vi "Template - Error Handler.vi"(7 "Command (Check for Error)":T5=enum."Check", 8 "error in (no error)":errorcluster, 11 "QU Ref cluster":T4) -> (0 "error out":errorcluster)   [LabVIEW 2012]
doc: "This VI is the main VI for the error module. This VI will shutdown the application cleanly if an error occurs.\n\nThe errors can then be reported back."
uses:
  Navistar Library/Controls/TypeDef_Error_Command_enum.ctl
  TypeDef - Template - Q1 Ref.ctl
  TypeDef - Template - Queue1 Data Enum.ctl
  TypeDef - Template - Q2 Ref.ctl
  TypeDef - Template - Queue2 Data Enum.ctl
  TypeDef - Template - UEvent Ref.ctl
  TypeDef - Template - UEvent Data Enum.ctl
panel:
  # "Inputs"
  # "Outputs"
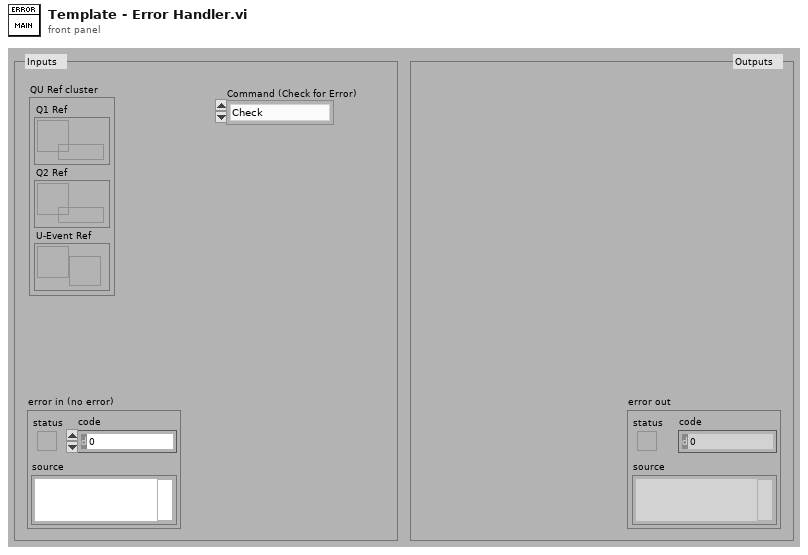
[diagram p1: front panel]
types:
  T1 = typedef "TypeDef - Template - Q1 Ref.ctl" = refnum<queue>
  T2 = typedef "TypeDef - Template - Q2 Ref.ctl" = refnum<queue>
  T3 = typedef "TypeDef - Template - UEvent Ref.ctl" = refnum<user-event>
  T4 = cluster{"Q1 Ref":T1, "Q2 Ref":T2, "U-Event Ref":T3}
  T5 = typedef "TypeDef_Error_Command_enum.ctl" = enum16{"Init", "Check", "Report"}
  T6 = typedef "TypeDef - Template - UEvent Data Enum.ctl" = enum16{"User Event", "Stop"}
  T7 = typedef "TypeDef - Template - Queue2 Data Enum.ctl" = enum16{"Queue Enum", "Change RPM", "Stop"}
  T8 = typedef "TypeDef - Template - Queue1 Data Enum.ctl" = enum16{"Queue Enum", "Get Time Data", "Check Time", "Stop"}
  T9 = typedef "TypeDef - UEvent Ref.ctl" = refnum<user-event>
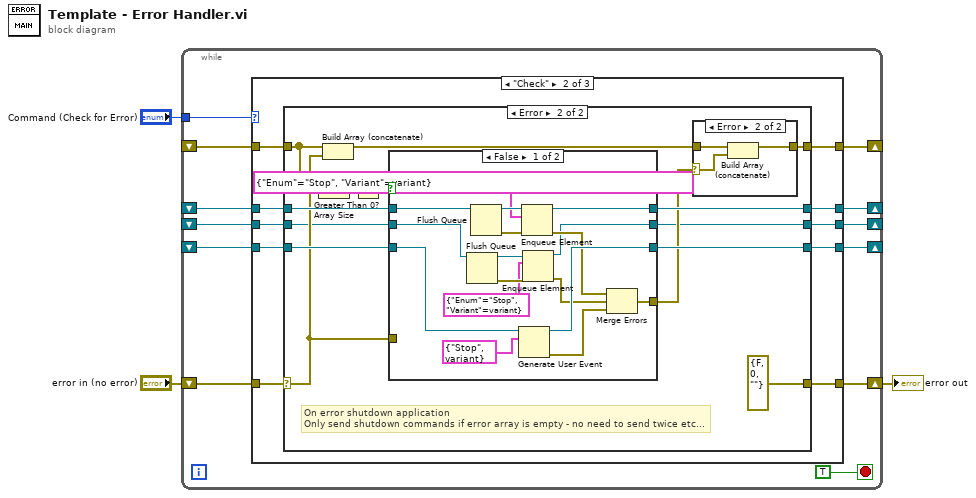
[diagram p0: block diagram]
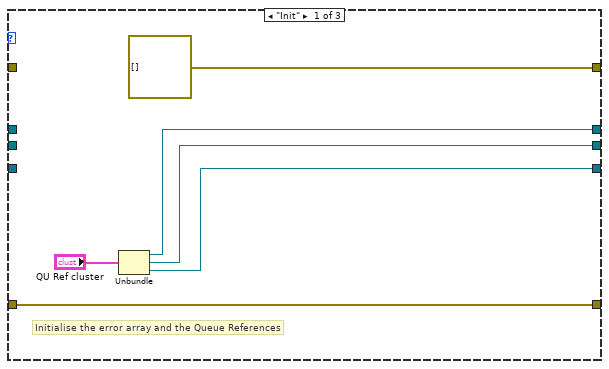
[diagram p2: hidden frame]
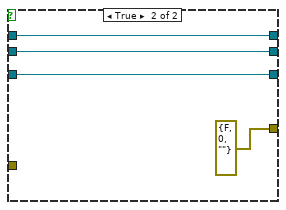
[diagram p4: hidden frame]
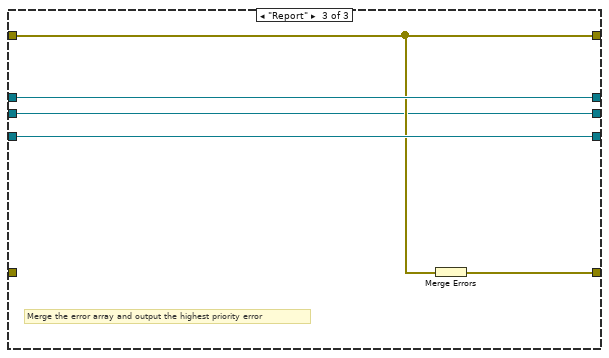
[diagram p6: hidden frame]
diagram:
  n1 = while {
    shift-right: [w14] -> w2
    shift-left: "error in (no error)" -> [w15]
    tunnel: "Command (Check for Error)" -> [w12]
    shift-right: [w11] -> _
    shift-left: _ -> [w9]
    shift-right: [w10] -> _
    shift-left: _ -> [w8]
    shift-right: [w7] -> _
    shift-left: _ -> [w6]
    shift-right: [w5] -> _
    shift-left: _ -> [w4]
    stop <- TRUE stop-if-true
    n2 = case shown="\"Check\"" w12 {
      tunnel: w15 -> [w21 w31 _]
      tunnel: [w21 w30 w77] -> w14
      tunnel: [w19 w27 w80] -> w11
      tunnel: [w18 w26 w79] -> w10
      tunnel: w9 -> [_ w29 w80]
      tunnel: w8 -> [_ w28 w79]
      tunnel: [errorcluster[] [] w24 w78] -> w7
      tunnel: w6 -> [_ w25 w78]
      tunnel: [w17 w22 w76] -> w5
      tunnel: w4 -> [_ w23 w76]
      frame "Init" {
        # "Initialise the error array and the Queue References"
        n3 = Unbundle("QU Ref cluster") -> ("Q1 Ref"=w19:T1, "Q2 Ref"=w17:T2, "U-Event Ref"=w18:T3)
      }
      frame "Check" {
        n4 = case shown="Error" w31 {
          selector: w31 -> [w36 w46]
          tunnel: [w36 errorcluster {"status"=FALSE, "code"=0, "source"=""} ("error IO")] -> w30
          tunnel: w29 -> [w35 w50]
          tunnel: w28 -> [w34 w48]
          tunnel: [w35 w49] -> w27
          tunnel: [w34 w47] -> w26
          tunnel: w25 -> [w33 w41]
          tunnel: [w33 w43] -> w24
          tunnel: w23 -> [w32 w38]
          tunnel: [w32 w37] -> w22
          frame No Error {
            # "No error - do nothing"
          }
          frame Error {
            # "On error shutdown application\nOnly send shutdown commands if error array is empty - no need to send twice etc..."
            n5 = Array Size(array=w41) -> (size(s)=w40:i32)
            n6 = Build Array (concatenate)(w41, w46) -> (w42:errorcluster[])
            n7 = Greater Than 0?(x=w40) -> (x > 0?=w39:bool)
            n8 = case shown="False" w39 {
              tunnel: w50 -> [w66 w71]
              tunnel: [w65 w71] -> w49
              tunnel: w48 -> [w63 w70]
              tunnel: [w62 w70] -> w47
              tunnel: w46 -> [_ _]
              tunnel: [w59 errorcluster {"status"=FALSE, "code"=0, "source"=""} ("error out")] -> w44
              tunnel: w38 -> [w56 w68]
              tunnel: [w54 w68] -> w37
              frame False {
                n9 = Flush Queue(queue=w56) -> (queue out=w55:T2, error out=w57:errorcluster)  [unwired: 1 in, 1 out]
                n10 = Flush Queue(queue=w66) -> (queue out=w67:T1, error out=w64:errorcluster)  [unwired: 1 in, 1 out]
                n11 = Generate User Event(user event=w63, event data cluster=cluster{"Data Type":T6, "Data":variant} {"Data Type"=enum."Stop", "Data"=variant} ("event data")) -> (user event out=w62:T9, error out=w60:errorcluster)  [unwired: 1 in]
                n12 = Enqueue Element(queue=w67, element=cluster{"Enum":T8, "Variant":variant} {"Enum"=enum."Stop", "Variant"=variant}, error in (no error)=w64) -> (queue out=w65:T1, error out=w61:errorcluster)  [unwired: 1 in, 1 out]
                n13 = Enqueue Element(queue=w55, element=cluster{"Enum":T7, "Variant":variant} {"Enum"=enum."Stop", "Variant"=variant}, error in (no error)=w57) -> (queue out=w54:T2, error out=w53:errorcluster)  [unwired: 1 in, 1 out]
                n14 = Merge Errors(w61, w53, w60) -> (w59:errorcluster)
              }
              frame True {
              }
            }
            n15 = case shown="Error" w44 {
              selector: w44 -> [_ w73]
              tunnel: w42 -> [w72 w75]
              tunnel: [w72 w74] -> w43
              frame No Error {
              }
              frame Error {
                n16 = Build Array (concatenate)(w75, w73) -> (w74:errorcluster[])
              }
            }
          }
        }
      }
      frame "Report" {
        # "Merge the error array and output the highest priority error"
        n17 = Merge Errors(w78) -> (w77:errorcluster)
      }
    }
  }
  "error out" <- w2
